vi "Execute.GetProfilePath.vi"(8 "error in (no error)":errorcluster, 11 "Profiles":refnum<vi>) -> (0 "error out":errorcluster, 3 "Path":path)   [LabVIEW 2013, in "Simple Sequence Editor.lvlib"]
uses:
  Simple Sequence Editor.lvlib
  NationalInstruments.VeriStand.Internal
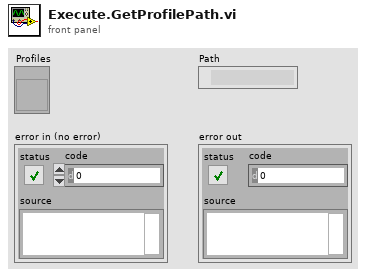
[diagram p1: front panel]
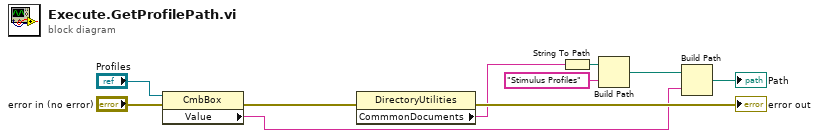
[diagram p0: block diagram]
diagram:
  n1 = property class="CmbBox"(reference="Profiles", error in="error in (no error)") -> (error out=w7:errorcluster, "Value"=w1:string)  [unwired: 1 out]
  n2 = property class="DirectoryUtilities"(error in=w7) -> (error out=→"error out":errorcluster, "CommmonDocuments"=w4:string)  [unwired: 1 in, 1 out]
  n3 = String To Path(string=w4) -> (path=w5:path)
  n4 = Build Path(base path=w5, name or relative path="Stimulus Profiles") -> (appended path=w9:path)
  n5 = Build Path(base path=w9, name or relative path=w1) -> (appended path=→"Path":path)
